vi "LoadMode.vi"(8 "error in (no error)":errorcluster, 10 "mode name":string, 11 "RSeries_CAM in":refnum<class "RSeries_CAM.lvclass">) -> (0 "error out":errorcluster, 2 "Success?":bool, 3 "RSeries_CAM out":refnum<class "RSeries_CAM.lvclass">)   [LabVIEW 2024, in "RSeries_CAM.lvlib" / "RSeries_CAM.lvclass"]
uses:
  RSeries_CAM.lvclass
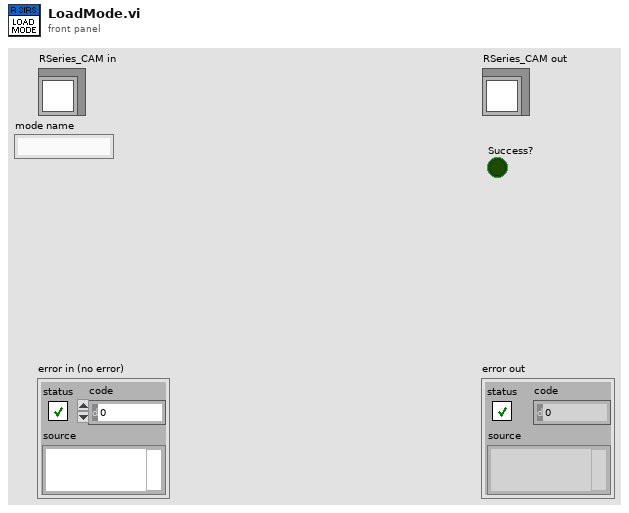
[diagram p1: front panel]
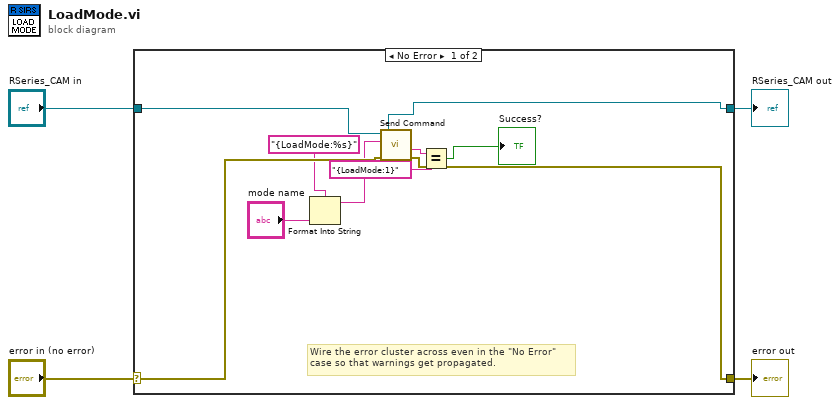
[diagram p0: block diagram]
diagram:
  n1 = case shown="No Error" "error in (no error)" {
    selector: "error in (no error)" -> [w12 w16]
    tunnel: [w11 w16] -> w3
    tunnel: [w13 w15] -> w1
    tunnel: "RSeries_CAM in" -> [w14 w15]
    frame No Error {
      # "Wire the error cluster across even in the \"No Error\"\ncase so that warnings get propagated."
      n2 = Format Into String(format string="{LoadMode:%s}" ("Command"), "mode name") -> (resulting string=w9:string)  [unwired: 2 in, 1 out]
      n3 = call "Send Command.vi"("error in (no error)"=w12, "Command"=w9, "RSeries_CAM in"=w14) -> ("error out"=w11:errorcluster, "Response"=w7:string, "RSeries_CAM out"=w13:refnum<class "RSeries_CAM.lvclass">)  [unwired: 5 in, 1 out]
      n4 = Equal?(x=w7, y="{LoadMode:1}") -> (x = y?=→"Success?":bool)
    }
    frame Error {
    }
  }
  "error out" <- w3
  "RSeries_CAM out" <- w1
